vi "init.vi"(8 "error in (no error)":errorcluster, 11 "UI Actor in":refnum<class "UI Actor.lvclass">) -> (0 "error out":errorcluster, 3 "UI Actor out":refnum<class "UI Actor.lvclass">)   [LabVIEW 2020, in "UI Actor.lvlib" / "UI Actor.lvclass"]
uses:
  UI Actor.lvclass
  C:/Program Files/National Instruments/LabVIEW 2020/vi.lib/ActorFramework/Actor/Actor.lvclass
  MENSAJE/MENSAJE.lvclass
  UI Actor.lvclass/UI Actor.ctl
  coffe actor/coffe actor.lvclass
  coffe actor/coffe actor.lvclass/coffe actor.ctl
  Soda Actor/Soda Actor.lvclass
  Soda Actor/Soda Actor.lvclass/Soda Actor.ctl
  USD Actor/USD Actor.lvclass
  USD Actor/USD Actor.lvclass/USD Actor.ctl
  MXN actor/MXN actor.lvclass
  MXN actor/MXN actor.lvclass/MXN actor.ctl
  MENSAJE/MENSAJE.lvclass/MENSAJE.ctl
  Read Monedas.vi
  Read Sub Panel coin.vi
  Read Productos.vi
  Read Sub Panel Prod.vi
  Read Sub Panel mensaje.vi
  <vilib>/ActorFramework/Actor/Actor.lvclass
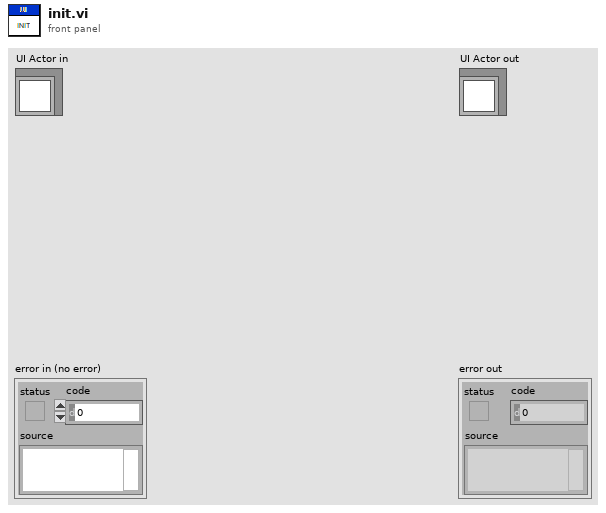
[diagram p1: front panel]
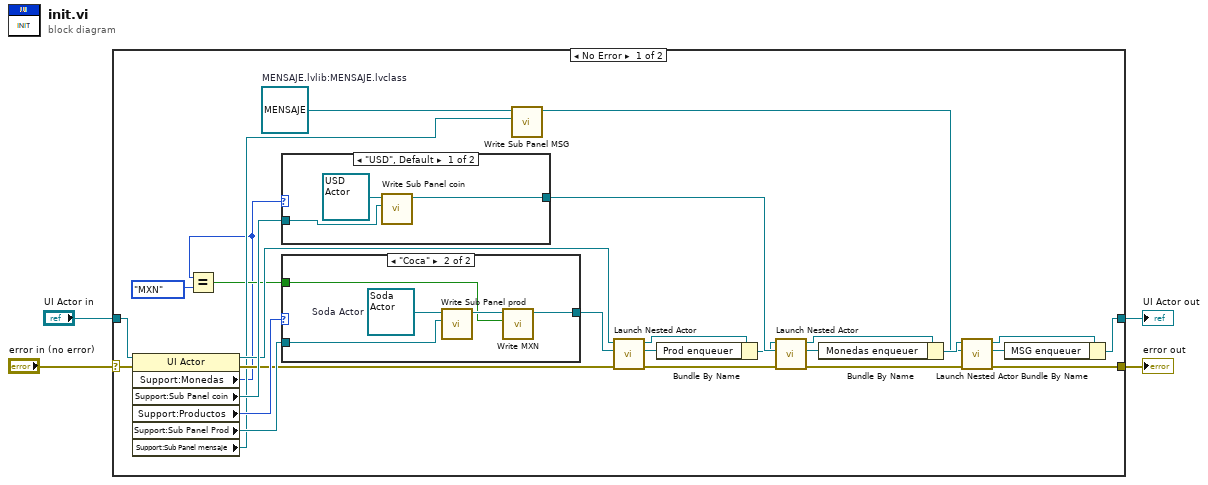
[diagram p0: block diagram]
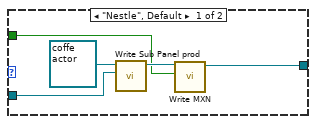
[diagram p2: hidden frame]
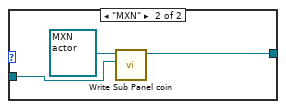
[diagram p3: hidden frame]
diagram:
  n1 = case shown="No Error" "error in (no error)" {
    selector: "error in (no error)" -> [w31 w49]
    tunnel: [w15 w49] -> w3
    tunnel: [w12 w48] -> w1
    tunnel: "UI Actor in" -> [w30 w48]
    frame No Error {
      w10 = refnum<class "MENSAJE.lvclass"> refnum  # MENSAJE.lvlib:MENSAJE.lvclass
      n2 = property class="UI Actor"(reference=w30, error in=w31) -> (reference out=w18:refnum<class "UI Actor.lvclass">, error out=w21:errorcluster, "Support:Monedas"=w5:enum16{"USD", "MXN"}, "Support:Sub Panel coin"=w25:refnum<vi>, "Support:Productos"=w24:enum16{"Nestle", "Coca"}, "Support:Sub Panel Prod"=w23:refnum<vi>, "Support:Sub Panel mensaje"=w9:refnum<vi>)
      n3 = Equal?(x=w5, y=enum16{"USD", "MXN"}."MXN" ("x")) -> (x = y?=w7:bool)
      n4 = case shown="\"USD\", Default" w5 {
        tunnel: [w43 w46] -> w28
        tunnel: w25 -> [w42 w45]
        frame "USD", Default {
          n5 = call "Write Sub Panel coin.vi"("Sub Panel coin"=w42, "USD Actor in"=refnum<class "USD Actor.lvclass"> refnum ("USD Actor.lvlib:USD Actor.lvclass")) -> ("USD Actor out"=w43:refnum<class "USD Actor.lvclass">)  [unwired: 8 in, 1 out]
        }
        frame "MXN" {
          n6 = call "Write Sub Panel coin.vi"("Sub Panel coin"=w45, "MXN actor in"=refnum<class "MXN actor.lvclass"> refnum ("MXN actor.lvlib:MXN actor.lvclass")) -> ("MXN actor out"=w46:refnum<class "MXN actor.lvclass">)  [unwired: 8 in, 1 out]
        }
      }
      n7 = case shown="\"Coca\"" w24 {
        tunnel: [w33 w38] -> w20
        tunnel: w23 -> [w35 w40]
        tunnel: w7 -> [w32 w37]
        frame "Nestle", Default {
          n8 = call "Write Sub Panel prod.vi"("Sub Panel prod"=w35, "coffe actor in"=refnum<class "coffe actor.lvclass"> refnum ("coffe actor.lvlib:coffe actor.lvclass")) -> ("coffe actor out"=w34:refnum<class "coffe actor.lvclass">)  [unwired: 8 in, 1 out]
          n9 = call "Write MXN.vi"("MXN"=w32, "coffe actor in"=w34) -> ("coffe actor out"=w33:refnum<class "coffe actor.lvclass">)  [unwired: 8 in, 1 out]
        }
        frame "Coca" {
          w41 = refnum<class "Soda Actor.lvclass"> refnum  # Soda Actor
          n10 = call "Write Sub Panel prod.vi"("Sub Panel prod"=w40, "Soda Actor in"=w41) -> ("Soda Actor out"=w39:refnum<class "Soda Actor.lvclass">)  [unwired: 8 in, 1 out]
          n11 = call "Write MXN.vi"("MXN"=w37, "Soda Actor in"=w39) -> ("Soda Actor out"=w38:refnum<class "Soda Actor.lvclass">)  [unwired: 8 in, 1 out]
        }
      }
      n12 = call "Write Sub Panel MSG.vi"("Sub Panel MSG"=w9, "MENSAJE in"=w10) -> ("MENSAJE out"=w8:refnum<class "MENSAJE.lvclass">)  [unwired: 8 in, 1 out]
      n13 = call <vilib>:"Launch Nested Actor.vi"("error in (no error)"=w21, "Nested Actor"=w20, "Caller Actor in"=w18) -> ("error out"=w22:errorcluster, "Nested Actor's Enqueuer"=w16:refnum<class "Message Enqueuer.lvclass">, "Caller Actor out"=w19:refnum<class "UI Actor.lvclass">)  [unwired: 6 in]
      n14 = Bundle By Name(cluster=w19, "Prod enqueuer"=w16) -> (w17:refnum<class "UI Actor.lvclass">)
      n15 = call <vilib>:"Launch Nested Actor.vi"("error in (no error)"=w22, "Nested Actor"=w28, "Caller Actor in"=w17) -> ("error out"=w29:errorcluster, "Nested Actor's Enqueuer"=w26:refnum<class "Message Enqueuer.lvclass">, "Caller Actor out"=w27:refnum<class "UI Actor.lvclass">)  [unwired: 6 in]
      n16 = Bundle By Name(cluster=w27, "Monedas enqueuer"=w26) -> (w14:refnum<class "UI Actor.lvclass">)
      n17 = call <vilib>:"Launch Nested Actor.vi"("error in (no error)"=w29, "Nested Actor"=w8, "Caller Actor in"=w14) -> ("error out"=w15:errorcluster, "Nested Actor's Enqueuer"=w11:refnum<class "Message Enqueuer.lvclass">, "Caller Actor out"=w13:refnum<class "UI Actor.lvclass">)  [unwired: 6 in]
      n18 = Bundle By Name(cluster=w13, "MSG enqueuer"=w11) -> (w12:refnum<class "UI Actor.lvclass">)
    }
    frame Error {
    }
  }
  "error out" <- w3
  "UI Actor out" <- w1
